vi "SSC Digital Write Sequencer Flag.vi"(0 "Digital SSC in":T1[](array[typedef]), 5 "Sequencer Flag":string(combo)="seqflag0", 7 "State":bool=TRUE caption="State (T)", 11 "error in":errorcluster) -> (4 "Digital SSC out":T1[](array[typedef]), 15 "error out":errorcluster)   [LabVIEW 2020]
doc: "Writes the state of a pattern sequencer flag on the device(s) connected to the specified pin(s) and pin group(s). Use pattern sequencer flags to coordinate execution between the pattern sequencer and a runtime test program."
uses:
  SSC Digital.ctl
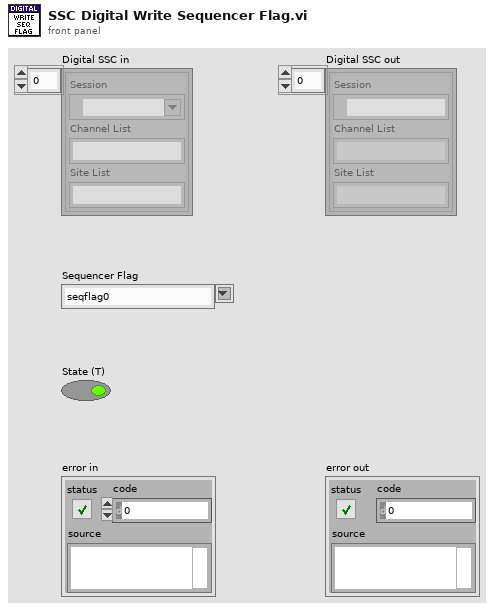
[diagram p1: front panel]
types:
  T1 = typedef "SSC Digital.ctl" = cluster{"Session":refnum<k15>, "Channel List":string, "Site List":string}
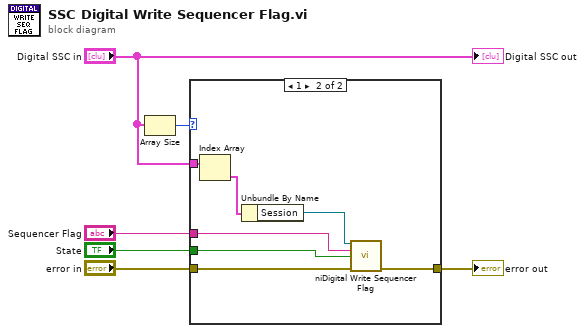
[diagram p0: block diagram]
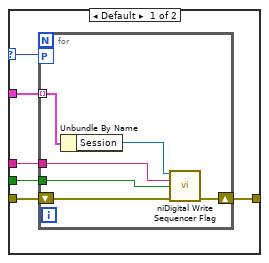
[diagram p2: hidden frame]
diagram:
  n1 = Array Size(array="Digital SSC in") -> (size(s)=w2:i32)
  n2 = case shown="1" w2 {
    selector: w2 -> [w8 _]
    tunnel: "Sequencer Flag" -> [w12 w25]
    tunnel: "State" -> [w11 w24]
    tunnel: "error in" -> [w10 w23]
    tunnel: [w9 w22] -> w3
    tunnel: "Digital SSC in" -> [w7 w21]
    frame Default {
      n3 = for {
        tunnel: w7 -> [w18] mode=indexing
        tunnel: w12 -> [w14]
        tunnel: w11 -> [w13]
        workers-P: w8 -> [_]
        shift-right: [w16] -> w9
        shift-left: w10 -> [w17]
        n4 = Unbundle By Name(w18) -> ("Session"=w15:refnum<k15>)
        n5 = call <instrlib>:"niDigital Write Sequencer Flag.vi"("instrument handle"=w15, "sequencer flag"=w14, "state (T)"=w13, "error in"=w17) -> ("error out"=w16:errorcluster)  [unwired: 10 in, 1 out]
      }
    }
    frame 1 {
      n6 = Index Array(array=w21) -> (element=w19:T1)  [unwired: 1 in]
      n7 = Unbundle By Name(w19) -> ("Session"=w20:refnum<k15>)
      n8 = call <instrlib>:"niDigital Write Sequencer Flag.vi"("instrument handle"=w20, "sequencer flag"=w25, "state (T)"=w24, "error in"=w23) -> ("error out"=w22:errorcluster)  [unwired: 10 in, 1 out]
    }
  }
  "error out" <- w3
  "Digital SSC out" <- "Digital SSC in"
